vi "Initialize Resource Config-Single.vi"(8 "error in":errorcluster, 11 "Initialize resource Config - Single":T1={"Resource name"="", "Voltage/current level"=0.0, "Voltage/current level range"=0.0, "Voltage/current limit range"=0.0, "Voltage/current limit low"=0.0, "Voltage/current limit high"=inf, "Output function"=1007, "Sense"=1009, "Transient response"=1038, "Voltage/current gain bandwidth"=0.0, "Voltage/current compensation frequency"=0.0, "Voltage/current pole-zero ratio"=0.0, "DUT set-up time"=0.0, "Limit symmetry"=enum."Symmetric"} {"Transient response" items=["Slow"=1041, "Normal"=1038, "Fast"=1039, "Custom"=1042]; "Sense" items=["Local"=1008, "Remote"=1009]; "Output function" items=["DC Voltage"=1006, "DC Current"=1007, "Pulse Voltage"=1049, "Pulse Current"=1050]; "Voltage/current limit high" format="%#_6p"; "Voltage/current limit low" format="%#_6p"; "Voltage/current limit range" format="%#_6p"}) -> (0 "error out":errorcluster, 2 "channel name":string, 3 "instrument handle out":refnum<k15>)   [LabVIEW 2021]
doc: "Initalize the source and load resource in single channel configuration."
uses:
  controls/Initialize Resource Config-Single.ctl
  <instrlib>/niDCPower/nidcpower.llb/niDCPower Source Mode.ctl
  <instrlib>/niDCPower/nidcpower.llb/niDCPower Wait For Event - Event.ctl
  <instrlib>/niDCPower/nidcpower.llb/niDCPower Get Channel Name From String.vi
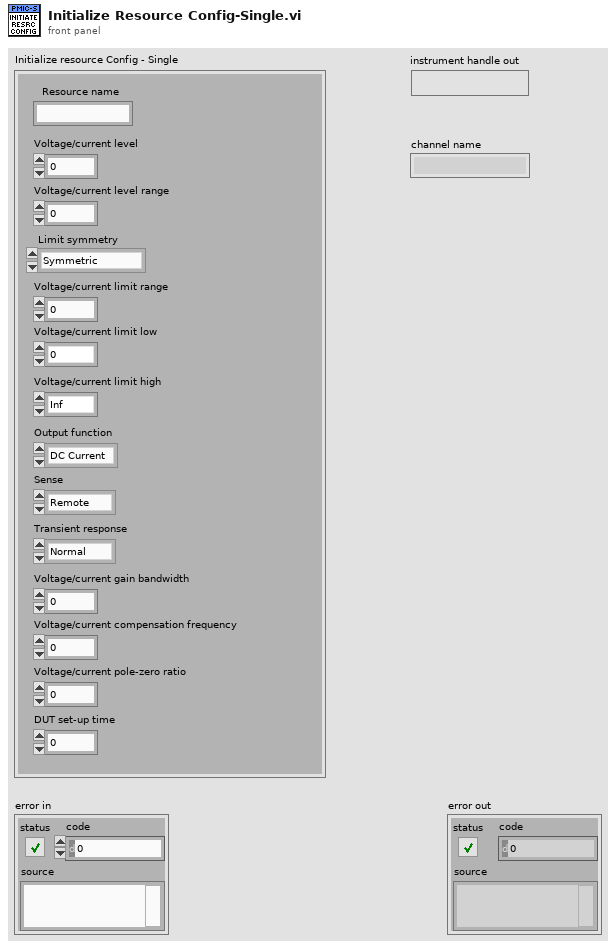
[diagram p1: front panel]
types:
  T1 = typedef "Initialize Resource Config-Single.ctl" = cluster{"Resource name":string, "Voltage/current level":dbl, "Voltage/current level range":dbl, "Voltage/current limit range":dbl, "Voltage/current limit low":dbl, "Voltage/current limit high":dbl, "Output function":i32, "Sense":i32, "Transient response":i32, "Voltage/current gain bandwidth":dbl, "Voltage/current compensation frequency":dbl, "Voltage/current pole-zero ratio":dbl, "DUT set-up time":dbl, "Limit symmetry":enum32{"Symmetric", "Asymmetric"}}
  T2 = typedef "niDCPower Wait For Event - Event.ctl" = i32
  T3 = typedef "niDCPower Source Mode.ctl" = i32
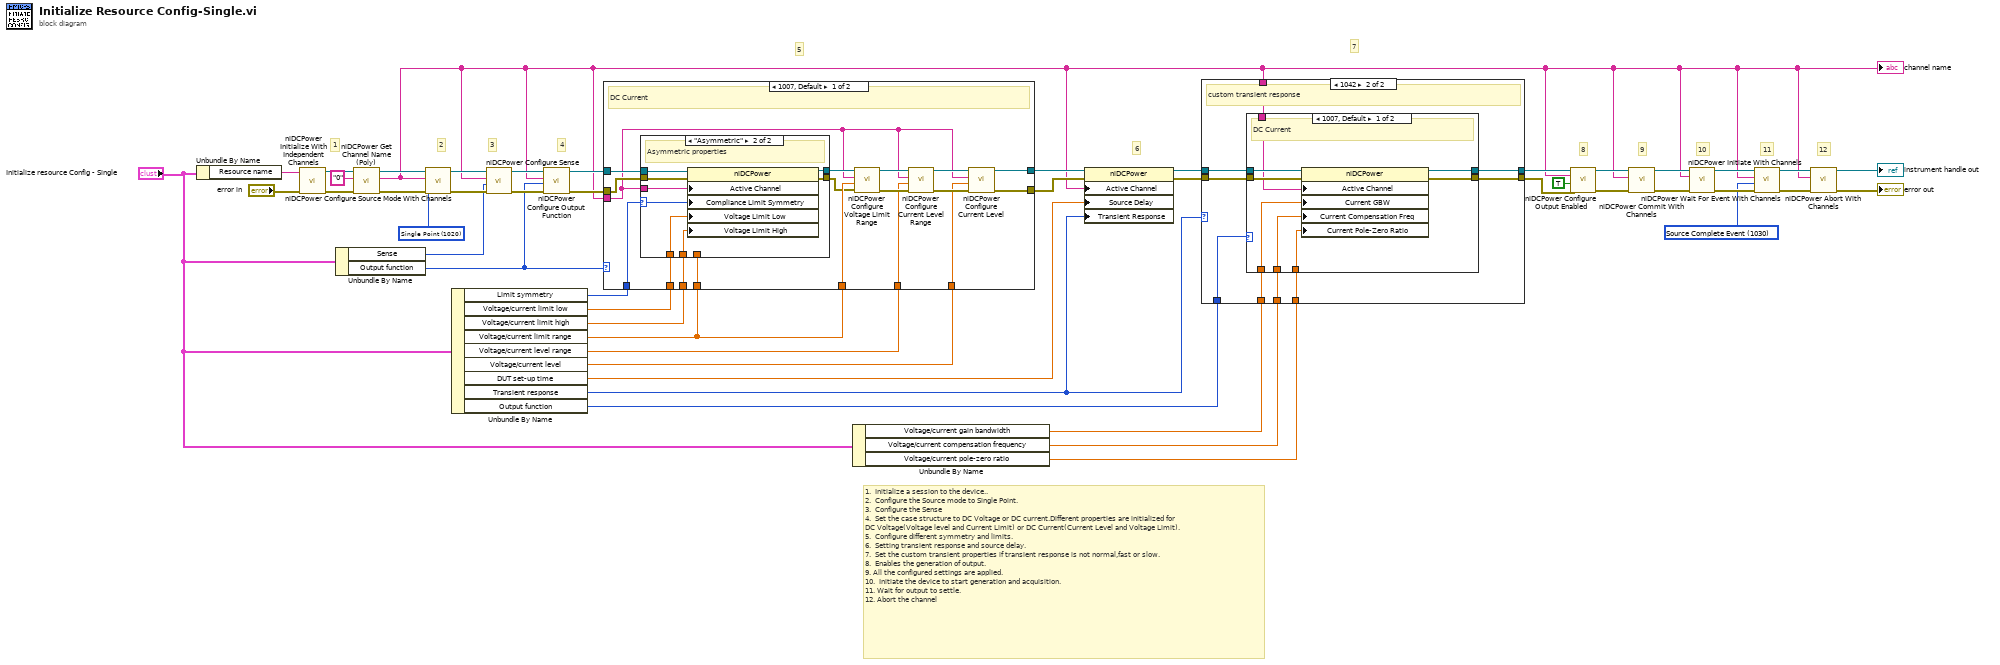
[diagram p0: block diagram]
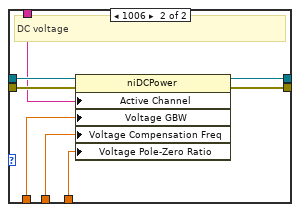
[diagram p3: hidden frame]
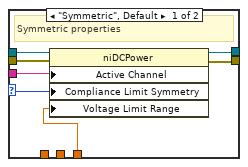
[diagram p4: hidden frame]
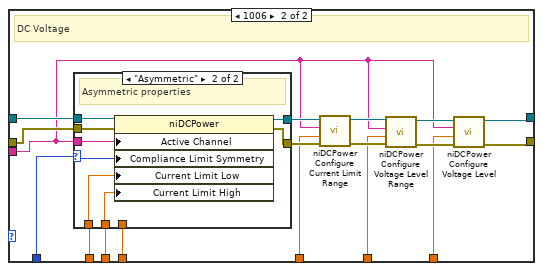
[diagram p5: hidden frame]
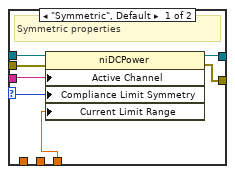
[diagram p6: hidden frame]
diagram:
  w11 = T2 1030 items=["Source Complete Event"=1030, "Measure Complete Event"=1031, "Sequence Iteration Complete Event"=1032, "Sequence Engine Done Event"=1033, "Pulse Complete Event"=1051, "Ready For Pulse Trigger Event"=1052] ("event")
  w43 = T3 1020 items=["Single Point"=1020, "Sequence"=1021] ("source mode")
  # "12"
  # "10"
  # "11"
  # "9"
  # "8"
  # "6"
  # "4"
  # "2"
  # "1.  Initialize a session to the device..\n2.  Configure the Source mode to Single Point.\n3.  Configure the Sense\n4.  Set the case structure to DC Voltage or DC current.Different properties are initialized for \nDC Voltage(Voltage level and Current Limit) or DC Current(Current Level and Voltage Limit). \n5.  Configure different symmetry and limits.\n6.  Setting transient response and source delay.\n7.  Set the custom transient properties if transient response is not normal,fast or slow.\n8.  Enables the generation of output.\n9. All the configured settings are applied.\n10.  Initiate the device to start generation and acquisition.\n11. Wait for output to settle.\n12. Abort the channel"
  # "7"
  # "5"
  # "1"
  # "3"
  n1 = Unbundle By Name("Initialize resource Config - Single") -> ("Resource name"=w7:string)
  n2 = call <instrlib>:"niDCPower Initialize With Independent Channels.vi"("error in (no error)"="error in", "resource name"=w7) -> ("error out"=w46:errorcluster, "instrument handle out"=w48:refnum<k15>)  [unwired: 8 in]
  n3 = Unbundle By Name("Initialize resource Config - Single") -> ("Sense"=w35:i32, "Output function"=w38:i32)
  n4 = call-poly <instrlib>:"niDCPower Get Channel Name (Poly).vi"("error in (no error)"=w46, "index"="0", "instrument handle"=w48) -> ("error out"=w45:errorcluster, "name"=w3:string, "instrument handle out"=w44:refnum<k15>)  [unwired: 6 in]
  "channel name" <- w3
  n5 = call <instrlib>:"niDCPower Configure Source Mode With Channels.vi"("error in (no error)"=w45, "source mode"=w43, "channel name"=w3, "instrument handle"=w44) -> ("error out"=w42:errorcluster, "instrument handle out"=w41:refnum<k15>)  [unwired: 6 in]
  n6 = Unbundle By Name("Initialize resource Config - Single") -> ("Limit symmetry"=w34:enum32{"Symmetric", "Asymmetric"}, "Voltage/current limit low"=w33:dbl, "Voltage/current limit high"=w32:dbl, "Voltage/current limit range"=w2:dbl, "Voltage/current level range"=w31:dbl, "Voltage/current level"=w30:dbl, "DUT set-up time"=w27:dbl, "Transient response"=w26:i32, "Output function"=w25:i32)
  n7 = call <instrlib>:"niDCPower Configure Sense.vi"("error in (no error)"=w42, "sense"=w35, "channel name"=w3, "instrument handle"=w41) -> ("error out"=w40:errorcluster, "instrument handle out"=w39:refnum<k15>)  [unwired: 6 in]
  n8 = call <instrlib>:"niDCPower Configure Output Function.vi"("error in (no error)"=w40, "output function"=w38, "channel name"=w3, "instrument handle"=w39) -> ("error out"=w36:errorcluster, "instrument handle out"=w37:refnum<k15>)  [unwired: 6 in]
  n9 = case shown="1007, Default" w38 {
    tunnel: w37 -> [w66 w99]
    tunnel: w36 -> [w65 w98]
    tunnel: w3 -> [w51 w84]
    tunnel: w34 -> [w50 w83]
    tunnel: w33 -> [w64 w97]
    tunnel: w32 -> [w63 w96]
    tunnel: w2 -> [w61 w89]
    tunnel: w31 -> [w57 w88]
    tunnel: w30 -> [w54 w87]
    tunnel: [w53 w86] -> w29
    tunnel: [w52 w85] -> w28
    tunnel: w2 -> [w49 w82]
    frame 1007, Default {
      # "DC Current"
      n10 = case shown="\"Asymmetric\"" w50 {
        selector: w50 -> [w73 w74]
        tunnel: w66 -> [w72 w81]
        tunnel: w65 -> [w71 w80]
        tunnel: w64 -> [_ w79]
        tunnel: w63 -> [_ w78]
        tunnel: [w69 w77] -> w62
        tunnel: [w68 w76] -> w60
        tunnel: w51 -> [w70 w75]
        tunnel: w49 -> [w67 _]
        frame "Symmetric", Default {
          # "Symmetric properties"
          n11 = property class="niDCPower"(reference=w72, error in=w71, "Active Channel"=w70, "Compliance Limit Symmetry"=w73, "Voltage Limit Range"=w67) -> (reference out=w69:refnum<k15>, error out=w68:errorcluster)
        }
        frame "Asymmetric" {
          # "Asymmetric properties"
          n12 = property class="niDCPower"(reference=w81, error in=w80, "Active Channel"=w75, "Compliance Limit Symmetry"=w74, "Voltage Limit Low"=w79, "Voltage Limit High"=w78) -> (reference out=w77:refnum<k15>, error out=w76:errorcluster)
        }
      }
      n13 = call <instrlib>:"niDCPower Configure Voltage Limit Range.vi"("error in (no error)"=w60, "voltage limit range"=w61, "channel name"=w51, "instrument handle"=w62) -> ("error out"=w59:errorcluster, "instrument handle out"=w58:refnum<k15>)  [unwired: 6 in]
      n14 = call <instrlib>:"niDCPower Configure Current Level Range.vi"("error in (no error)"=w59, "current level range"=w57, "channel name"=w51, "instrument handle"=w58) -> ("error out"=w56:errorcluster, "instrument handle out"=w55:refnum<k15>)  [unwired: 6 in]
      n15 = call <instrlib>:"niDCPower Configure Current Level.vi"("error in (no error)"=w56, "current level"=w54, "channel name"=w51, "instrument handle"=w55) -> ("error out"=w52:errorcluster, "instrument handle out"=w53:refnum<k15>)  [unwired: 6 in]
    }
    frame 1006 {
      # "DC Voltage"
      n16 = case shown="\"Asymmetric\"" w83 {
        selector: w83 -> [w103 w107]
        tunnel: w99 -> [w106 w114]
        tunnel: w98 -> [w105 w113]
        tunnel: w97 -> [_ w112]
        tunnel: w96 -> [_ w111]
        tunnel: [w100 w110] -> w95
        tunnel: [w101 w109] -> w94
        tunnel: w84 -> [w104 w108]
        tunnel: w82 -> [w102 _]
        frame "Symmetric", Default {
          # "Symmetric properties"
          n17 = property class="niDCPower"(reference=w106, error in=w105, "Active Channel"=w104, "Compliance Limit Symmetry"=w103, "Current Limit Range"=w102) -> (reference out=w101:refnum<k15>, error out=w100:errorcluster)
        }
        frame "Asymmetric" {
          # "Asymmetric properties"
          n18 = property class="niDCPower"(reference=w114, error in=w113, "Active Channel"=w108, "Compliance Limit Symmetry"=w107, "Current Limit Low"=w112, "Current Limit High"=w111) -> (reference out=w109:refnum<k15>, error out=w110:errorcluster)
        }
      }
      n19 = call <instrlib>:"niDCPower Configure Current Limit Range.vi"("error in (no error)"=w95, "current limit range"=w89, "channel name"=w84, "instrument handle"=w94) -> ("error out"=w93:errorcluster, "instrument handle out"=w92:refnum<k15>)  [unwired: 6 in]
      n20 = call <instrlib>:"niDCPower Configure Voltage Level Range.vi"("error in (no error)"=w93, "voltage level range"=w88, "channel name"=w84, "instrument handle"=w92) -> ("error out"=w91:errorcluster, "instrument handle out"=w90:refnum<k15>)  [unwired: 6 in]
      n21 = call <instrlib>:"niDCPower Configure Voltage Level.vi"("error in (no error)"=w91, "voltage level"=w87, "channel name"=w84, "instrument handle"=w90) -> ("error out"=w85:errorcluster, "instrument handle out"=w86:refnum<k15>)  [unwired: 6 in]
    }
  }
  n22 = Unbundle By Name("Initialize resource Config - Single") -> ("Voltage/current gain bandwidth"=w10:dbl, "Voltage/current compensation frequency"=w9:dbl, "Voltage/current pole-zero ratio"=w8:dbl)
  n23 = property class="niDCPower"(reference=w29, error in=w28, "Active Channel"=w3, "Source Delay"=w27, "Transient Response"=w26) -> (reference out=w24:refnum<k15>, error out=w23:errorcluster)
  n24 = case shown="1042" w26 {
    tunnel: w25 -> [_ w125]
    tunnel: w24 -> [w115 w124]
    tunnel: w23 -> [w116 w123]
    tunnel: w10 -> [_ w122]
    tunnel: w9 -> [_ w121]
    tunnel: w8 -> [_ w120]
    tunnel: w3 -> [_ w119]
    tunnel: [w115 w118] -> w22
    tunnel: [w116 w117] -> w21
    frame Default {
      # "Normal, fast and slow transient"
    }
    frame 1042 {
      # "custom transient response"
      n25 = case shown="1007, Default" w125 {
        tunnel: w124 -> [w133 w141]
        tunnel: w123 -> [w132 w140]
        tunnel: w122 -> [w131 w139]
        tunnel: w121 -> [w130 w138]
        tunnel: w120 -> [w129 w137]
        tunnel: w119 -> [w128 w136]
        tunnel: [w127 w135] -> w118
        tunnel: [w126 w134] -> w117
        frame 1007, Default {
          # "DC Current"
          n26 = property class="niDCPower"(reference=w133, error in=w132, "Active Channel"=w128, "Current GBW"=w131, "Current Compensation Freq"=w130, "Current Pole-Zero Ratio"=w129) -> (reference out=w127:refnum<k15>, error out=w126:errorcluster)
        }
        frame 1006 {
          # "DC voltage"
          n27 = property class="niDCPower"(reference=w141, error in=w140, "Active Channel"=w136, "Voltage GBW"=w139, "Voltage Compensation Freq"=w138, "Voltage Pole-Zero Ratio"=w137) -> (reference out=w135:refnum<k15>, error out=w134:errorcluster)
        }
      }
    }
  }
  n28 = call <instrlib>:"niDCPower Configure Output Enabled.vi"("error in (no error)"=w21, "output enabled"=TRUE, "channel name"=w3, "instrument handle"=w22) -> ("error out"=w19:errorcluster, "instrument handle out"=w18:refnum<k15>)  [unwired: 6 in]
  n29 = call <instrlib>:"niDCPower Commit With Channels.vi"("error in (no error)"=w19, "channel name"=w3, "instrument handle"=w18) -> ("error out"=w17:errorcluster, "instrument handle out"=w16:refnum<k15>)  [unwired: 7 in]
  n30 = call <instrlib>:"niDCPower Initiate With Channels.vi"("error in (no error)"=w17, "channel name"=w3, "instrument handle"=w16) -> ("error out"=w15:errorcluster, "instrument handle out"=w14:refnum<k15>)  [unwired: 7 in]
  n31 = call <instrlib>:"niDCPower Wait For Event With Channels.vi"("error in (no error)"=w15, "event"=w11, "channel name"=w3, "instrument handle"=w14) -> ("error out"=w13:errorcluster, "instrument handle out"=w12:refnum<k15>)  [unwired: 6 in]
  n32 = call <instrlib>:"niDCPower Abort With Channels.vi"("error in (no error)"=w13, "channel name"=w3, "instrument handle"=w12) -> ("error out"=→"error out":errorcluster, "instrument handle out"=→"instrument handle out":refnum<k15>)  [unwired: 7 in]
